vi "Color Image.vi"() -> ()   [LabVIEW 2016]
uses:
  graph_utilities.lvclass
panel:
  in  "CET":T1(ring)
  in  "Test Image":enum16{"Bitches Brew", "Color Map"}(ring)
  in  "Color Map":T2(ring)
  out "Image":u32[][](graph)
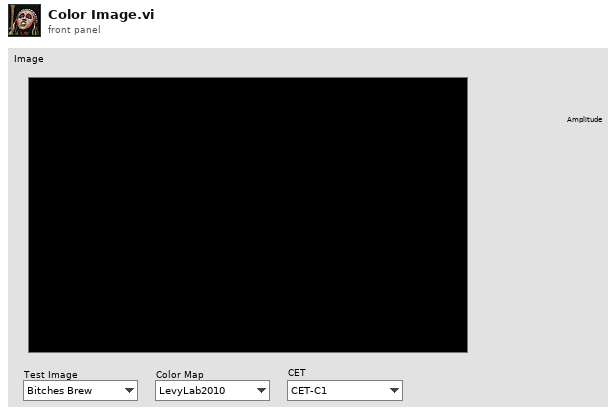
[diagram p1: front panel]
types:
  T1 = enum16{"CET-C1", "CET-C1s", "CET-C2", "CET-C2s", "CET-C3", "CET-C3s", "CET-C4", "CET-C4s", "CET-C5", "CET-C5s", "CET-C6", "CET-C6s", "CET-C7", "CET-C7s", "CET-CBC1", "CET-CBC2", "CET-CBD1", "CET-CBL1", "CET-CBL2", "CET-D01", "CET-D01A", "CET-D02", "CET-D03", "CET-D04", "CET-D06", "CET-D07", "CET-D08", "CET-D09", "CET-D10", "CET-D11", "CET-D12", "CET-D13", "CET-I1", "CET-I2", "CET-I3", "CET-L01", "CET-L02", "CET-L03", "CET-L04", "CET-L05", "CET-L06", "CET-L07", "CET-L08", "CET-L09", "CET-L10", "CET-L11", "CET-L12", "CET-L13", "CET-L14", "CET-L15", "CET-L16", "CET-L17", "CET-L18", "CET-L19", "CET-L20", "CET-R1", "CET-R2", "CET-R3", "CET-R4"}
  T2 = enum16{"LevyLab2010", "Inferno", "kindlmann", "plasma", "viridis", "CET"}
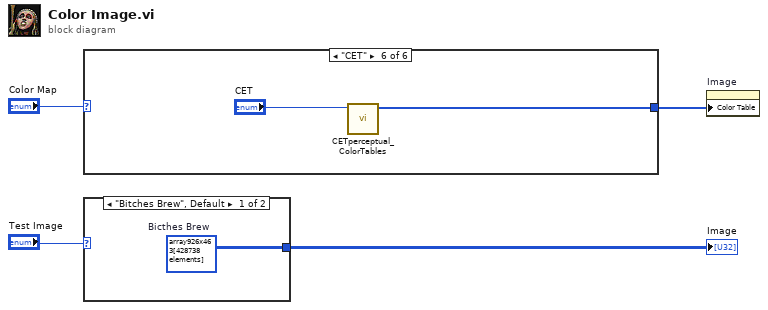
[diagram p0: block diagram]
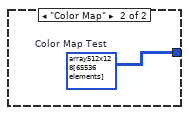
[diagram p2: hidden frame]
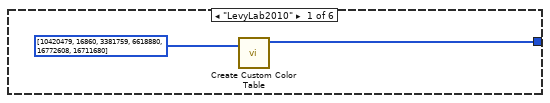
[diagram p3: hidden frame]
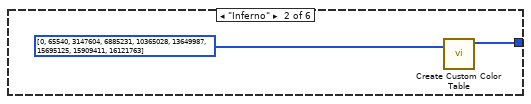
[diagram p4: hidden frame]
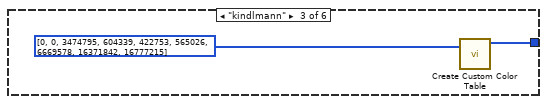
[diagram p5: hidden frame]
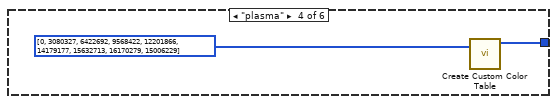
[diagram p6: hidden frame]
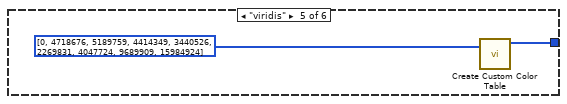
[diagram p7: hidden frame]
diagram:
  n1 = case shown="\"CET\"" "Color Map" {
    tunnel: [w5 w8 w10 w12 w14 w15] -> w1
    frame "LevyLab2010" {
      n2 = call "Create Custom Color Table.vi"("Colors []"=u32[] [10420479, 16860, 3381759, 6618880, 16772608, 16711680]) -> ("Color Tbl"=w5:u32[])  [unwired: 1 in, 3 out]
    }
    frame "Inferno" {
      n3 = call "Create Custom Color Table.vi"("Colors []"=u32[] [0, 65540, 3147604, 6885231, 10365028, 13649987, 15695125, 15909411, 16121763]) -> ("Color Tbl"=w8:u32[])  [unwired: 1 in, 3 out]
    }
    frame "kindlmann" {
      n4 = call "Create Custom Color Table.vi"("Colors []"=u32[] [0, 0, 3474795, 604339, 422753, 565026, 6669578, 16371842, 16777215]) -> ("Color Tbl"=w10:u32[])  [unwired: 1 in, 3 out]
    }
    frame "plasma" {
      n5 = call "Create Custom Color Table.vi"("Colors []"=u32[] [0, 3080327, 6422692, 9568422, 12201866, 14179177, 15632713, 16170279, 15006229]) -> ("Color Tbl"=w12:u32[])  [unwired: 1 in, 3 out]
    }
    frame "viridis" {
      n6 = call "Create Custom Color Table.vi"("Colors []"=u32[] [0, 4718676, 5189759, 4414349, 3440526, 2269831, 4047724, 9689909, 15984924]) -> ("Color Tbl"=w14:u32[])  [unwired: 1 in, 3 out]
    }
    frame "CET" {
      n7 = call "CETperceptual_ColorTables.vi"("CET"="CET") -> ("Color Table"=w15:u32[])  [unwired: 7 in, 3 out]
    }
  }
  n8 = case shown="\"Bitches Brew\", Default" "Test Image" {
    tunnel: [w17 w18] -> w2
    frame "Bitches Brew", Default {
      w17 = u32[][] array926x463[428738 elements]  # Bicthes Brew
    }
    frame "Color Map" {
      w18 = u32[][] array512x128[65536 elements]  # Color Map Test
    }
  }
  "Image" <- w2
  n9 = property on="Image" class="IntGraph (strict)"("Color Table"=w1) -> ()  [unwired: 2 in, 2 out]
